vi "NIDMM_Close.vi"(8 "error in (no error)":errorcluster, 11 "instrument handle":refnum<k15>="NI_DMM") -> (0 "error out":errorcluster)   [LabVIEW 2015]
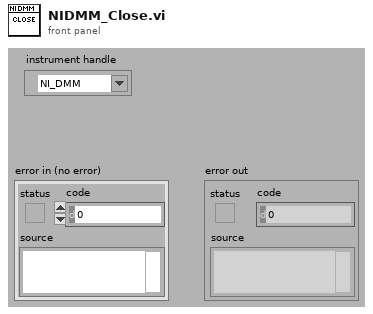
[diagram p1: front panel]
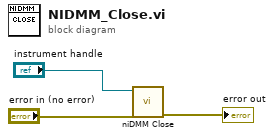
[diagram p0: block diagram]
diagram:
  n1 = call <instrlib>:"niDMM Close.vi"("error in (no error)"="error in (no error)", "instrument handle"="instrument handle") -> ("error out"=→"error out":errorcluster)  [unwired: 9 in]
